vi "observacao_queued.vi"() -> ()   [LabVIEW 2012, in "Shared_160.lvlib"] (continued)
                    n1067 = call "Trata PDA.vi"() -> ()  [unwired: 2 in]
                  }
                  frame True {
                    n1068 = call "Find ppctxt.vi"() -> ("Existe ppc.txt?"=w1386:bool, "ppc.txt Path"=w1385:path)  [unwired: 1 in]
                    n1069 = case shown="True" w1386 {
                      tunnel: w1385 -> [_ w1387]
                      frame False {
                      }
                      frame True {
                        # "limpa o arquivo ppc.txt"
                        n1070 = call "Wipe file.vi"("ppc path"=w1387) -> ()  [unwired: 2 out]
                      }
                    }
                  }
                }
              }
              frame #1 {
                n1071 = case shown="False" "Case Constant\n(See Context Help) 3" {
                  frame False {
                  }
                  frame True {
                    # "MUDANÇA:\nÉ necesário \nsubstituir as variáveis simuladas pelas do Sistema"
                    # "Simula os dados sendo alterados pela\nmovimentação do sistema"
                    n1072 = call "Data Table.vi"() -> ()  [unwired: 1 in]
                  }
                }
              }
              frame #2 {
                n1073 = case shown="True" "Case Constant\n(See Context Help) 4" {
                  frame False {
                  }
                  frame True {
                    # "Lê o arquivo padrão para o equip/o\nselecionado pelo PDA e grava o\narquivo ppcDisplay.htm adequado"
                    n1074 = call "Update Frame.vi"() -> ("Timeout"=w1390:u32)  [unwired: 2 in, 3 out]
                    n1075 = Wait Until Next ms Multiple(millisecond multiple=w1390) -> ()  [unwired: 1 out]
                  }
                }
              }
            }
          }
        }
        n1076 = global read "Global_Telescopio.vi" "Flag-Rotator"() -> (w83:bool)
        n1077 = case shown="True" w83 {
          frame False {
          }
          frame True {
            n1078 = local write "Setup, Pointing & Guiding"(T2."ROTATOR" ("Setup, Pointing & Guiding")) -> ()
          }
        }
      }
      frame #2 {
        n1079 = case shown="\"FOCUS\"" "Setup, Pointing & Guiding" {
          frame "POINTING", Default {
            n1080 = stacked-sequence {
              frame #0 {
                # "Clear Dados"
                n1081 = case shown="True" "BtPointObjClear" {
                  frame False {
                  }
                  frame True {
                    w1395 = ""
                    n1082 = local write "StrPointObjName"(w1395) -> ()
                    n1083 = local write "StrPointObjPMRA"(w1395) -> ()
                    n1084 = local write "StrPointObjPMDEC"(w1395) -> ()
                    n1085 = local write "StrPointObjRA"(w1395) -> ()
                    n1086 = local write "StrPointObjDEC"(w1395) -> ()
                    n1087 = local write "StrPointObjEpoch"(w1395) -> ()
                    n1088 = local write "StrPointTargetRA"(w1395) -> ()
                    n1089 = local write "StrPointTargetDEC"(w1395) -> ()
                  }
                }
                n1090 = local read "ChkCalLocal"() -> (w1392:bool)
                n1091 = case shown="False" w1392 {
                  selector: w1392 -> [w1394 _]
                  frame False {
                    # "Para de Piscar/Blink\no botão"
                    n1092 = property on="ChkCalLocal" class="Bool (strict)"("Blinking"=w1394) -> ()  [unwired: 2 in, 2 out]
                  }
                  frame True {
                  }
                }
              }
              frame #1 {
                w1402 = ""
                # "A forma como os mostradores da janela TARGET são carregados está indefinida.\nVamos colocar um botão SET ao lado do botão CLEAR na janela OBJECT.\nQuando o botão SET for pressionado, os mostradores da janela TARGET\nseriam calculados a partir dos valores da janela OBJECT."
                n1093 = local read "StrPointObjDEC"() -> (w1403:string)
                n1094 = local read "StrPointObjRA"() -> (w1404:string)
                n1095 = local read "StrPointObjPMDEC"() -> (w1396:string)
                n1096 = local read "StrPointObjPMRA"() -> (w1397:string)
                n1097 = Not Equal?(x=w1404, y=w1402) -> (x != y?=w1401:bool)
                n1098 = Not Equal?(x=w1403, y=w1402) -> (x != y?=w1400:bool)
                n1099 = local read "pressão atm"() -> (w1406:string)
                n1100 = local read "Temp amb"() -> (w1407:string)
                n1101 = local read "hum local"() -> (w1405:string)
                n1102 = And(x=w1401, y=w1400) -> (x .and. y?=w1398:bool)
                n1103 = And(x="BtPointPrecess", y=w1398) -> (x .and. y?=w1399:bool)
                n1104 = case shown="True" w1399 {
                  tunnel: w1404 -> [_ w1415]
                  tunnel: w1403 -> [_ w1414]
                  tunnel: w1407 -> [_ w1413]
                  tunnel: w1406 -> [_ w1412]
                  tunnel: w1405 -> [_ w1411]
                  tunnel: w1397 -> [_ w1410]
                  tunnel: w1396 -> [_ w1409]
                  frame False {
                  }
                  frame True {
                    n1105 = stacked-sequence {
                      tunnel: w1415 -> [w1449 _ _]
                      tunnel: w1414 -> [w1447 _ _]
                      tunnel: w1413 -> [w1457 _ _]
                      tunnel: w1412 -> [w1456 _ _]
                      tunnel: w1411 -> [w1455 _ _]
                      tunnel: w1410 -> [w1423 _ _]
                      tunnel: w1409 -> [w1422 _ _]
                      frame #0 {
                        # "PROCESSO PRECESSÃO"
                        # "MUDANÇA:\nVI Botao SET trocada por Botao Precess, eliminando entrada do Frame de coord. (Mean, Topo, Geo)"
                        n1106 = local read "ChkPointPrecessed"() -> (w1427:bool)
                        n1107 = call "Comma_to_Point.vi"("Lat_A"=w1455) -> ("Saída"=w1424:string)
                        n1108 = call "Comma_to_Point.vi"("Lat_A"=w1457) -> ("Saída"=w1426:string)
                        n1109 = call "Comma_to_Point.vi"("Lat_A"=w1456) -> ("Saída"=w1425:string)
                        n1110 = call "Comma_to_Point.vi"("Lat_A"=w1447) -> ("Saída"=w1442:string)
                        n1111 = call "Comma_to_Point.vi"("Lat_A"=w1449) -> ("Saída"=w1445:string)
                        n1112 = call "hms_rad.vi"("True = hora"=FALSE, "Texto Graus"=w1442) -> ("radianos"=w1441:dbl)  [unwired: 3 in]
                        n1113 = call "hms_rad.vi"("True = hora"=TRUE, "Texto Graus"=w1445) -> ("radianos"=w1444:dbl)  [unwired: 3 in]
                        n1114 = call "Arcsec to Rad_ String.vi"("VAR ARCSEC"=w1423) -> ("VAR RAD"=w1421:string)
                        n1115 = Number To Fractional String(use system decimal point (T)=FALSE, number=w1441, precision (6)=i16 9) -> (F-format string=w1430:string)  [unwired: 1 in]
                        n1116 = Number To Fractional String(use system decimal point (T)=FALSE, number=w1444, precision (6)=i16 9) -> (F-format string=w1431:string)  [unwired: 1 in]
                        n1117 = call "Arcsec to Rad_ String.vi"("VAR ARCSEC"=w1422) -> ("VAR RAD"=w1420:string)
                        n1118 = call "Botão Precess.vi"("AR"=w1431, "Precessed Coord."=w1427, "Dec"=w1430, "Temp local amb(K)"=w1426, "Pressao atm local (mB)"=w1425, "Hum rel local"=w1424, "Var RA"=w1421, "Var DEC"=w1420) -> ("RA"=w1459:dbl, "DEC"=w1416:dbl, "Hora Sideral (rad)"=w1458:dbl, "Dist. Zenital (rad)"=w1429:dbl, "Observed HA (radians)"=→"HA obs":dbl, "Massa de Ar"=w1428:dbl)  [unwired: 2 in]
                        "RA obs" <- w1459
                        "DEC obs" <- w1416
                        n1119 = local write "Zenital angle"(w1429) -> ()
                        n1120 = call "rad_hms.vi"("TRUE=HORA\nFALSE=GRAU"=FALSE ("TRUE=HORA\nFALSE=GRAU"), "Radiano"=w1416) -> ("Hora/Graus Texto Decimal"=w1437:string)  [unwired: 3 in]
                        n1121 = call "rad-graus.vi"("Radiano"=w1429) -> ("Graus"=w1454:dbl)
                        n1122 = Number To Fractional String(number=w1428, precision (6)=i16 3) -> (F-format string=→"Air Mass":string)  [unwired: 2 in]
                        n1123 = Number To Fractional String(number=w1454, precision (6)=i16 1) -> (F-format string=→"Zenital Angle":string)  [unwired: 2 in]
                        n1124 = call "rad_hms.vi"("TRUE=HORA\nFALSE=GRAU"=TRUE ("TRUE=HORA"), "Radiano"=w1459) -> ("Hora/Graus Texto Decimal"=w1439:string)  [unwired: 3 in]
                        n1125 = local write "StrPointTargetDEC"(w1437) -> ()
                        n1126 = local write "StrPointTargetRA"(w1439) -> ()
                        n1127 = disable-structure shown="Disabled" {
                          disable-tunnel: [w1463 _] -> _
                          disable-tunnel: w1459 -> [w1462 _]
                          disable-tunnel: w1458 -> [w1461 _]
                          disable-tunnel: w1416 -> [w1460 _]
                          frame Disabled {
                            n1128 = call "Hora_Limite.vi"("Asc Reta RA rad"=w1462, "Sideral Time rad"=w1461, "Declinação rad"=w1460) -> ("TO Tempo de Observação Horas"=w1463:dbl)  [unwired: 2 in]
                          }
                          frame Enabled {
                          }
                        }
                        n1129 = call "Novo_tempo_obs_inicial.vi"("TS"=w1458, "RA"=w1459, "DEC"=w1416) -> ("TO rad"=w1417:dbl)  [unwired: 7 in, 1 out]
                        n1130 = case shown="True" "TRUE=HORA\nFALSE=GRAU" {
                          frame False {
                          }
                          frame True {
                            # "Sincroniza hora do\nPC com GPS"
                            n1131 = call "About_Time.vi"() -> ()  [unwired: 1 in]
                          }
                        }
                        n1132 = call "rad_hms.vi"("TRUE=HORA\nFALSE=GRAU"=TRUE ("TRUE=HORA\nFALSE=GRAU"), "Radiano"=w1417) -> ("Hora/Graus Texto Decimal"=→"Tempo Obs":string)  [unwired: 3 in]
                      }
                      frame #1 {
                        # "Testa o ângulo zenital menor que 70º o led \"Working Area\" \naceso na cor verde se o ângulozenital menor que 70º e \nvermelho em caso cont rário."
                        n1133 = global read "Global_Telescopio.vi" "Piscar working area"() -> (w1470:bool)
                        n1134 = global read "Global_Telescopio.vi" "working area = VERDE"() -> (w1469:bool)
                        n1135 = global read "Global_Telescopio.vi" "ativar botão GO"() -> (w1467:bool)
                        n1136 = case shown="True" w1469 {
                          frame False {
                            # "False=Vermelho"
                            n1137 = local write "LedPointWorkArea"(FALSE ("LedPointWorkArea")) -> ()
                          }
                          frame True {
                            # "True=Verde"
                            "LedPointWorkArea" <- TRUE ("LedPointWorkArea")
                          }
                        }
                        n1138 = global write "Global_Telescopio.vi" "Botão GO = STOP"(FALSE ("Botão GO = STOP")) -> ()
                        n1139 = case shown="True" w1467 {
                          selector: w1467 -> [_ w1471]
                          frame False {
                          }
                          frame True {
                            n1140 = property on="BtTargetPoint" class="Bool"("Visible"=w1471) -> ()  [unwired: 2 in, 2 out]
                          }
                        }
                        n1141 = global write "Global_Telescopio.vi" "Piscar working area"(w1470) -> ()
                        n1142 = global read "Global_Telescopio.vi" "desativar botão GO"() -> (w1468:bool)
                        n1143 = case shown="True" w1468 {
                          selector: w1468 -> [_ w1473]
                          frame False {
                          }
                          frame True {
                            n1144 = Not(x=w1473) -> (.not. x?=w1472:bool)
                            n1145 = property on="BtTargetPoint" class="Bool"("Visible"=w1472) -> ()  [unwired: 2 in, 2 out]
                          }
                        }
                        n1146 = property on="LedPointWorkArea" class="Bool (strict)"("Visible"=TRUE ("Botão GO = STOP")) -> ()  [unwired: 2 in, 2 out]
                        n1147 = property on="LedPointing" class="Bool (strict)"("Visible"=FALSE) -> ()  [unwired: 2 in, 2 out]
                      }
                      frame #2 {
                        n1148 = global read "Global_Telescopio.vi" "CalDEC Local"() -> (w1481:dbl)
                        n1149 = global read "Global_Telescopio.vi" "CalAH Local"() -> (w1482:dbl)
                        n1150 = local read "ChkCalLocal"() -> (w1476:bool)
                        n1151 = Not Equal To 0?(x=w1482) -> (x != 0?=w1479:bool)
                        n1152 = Not Equal To 0?(x=w1481) -> (x != 0?=w1480:bool)
                        n1153 = Or(x=w1479, y=w1480) -> (x .or. y?=w1477:bool)
                        n1154 = And(x=w1476, y=w1477) -> (x .and. y?=w1478:bool)
                        n1155 = case shown="True" w1478 {
                          frame False {
                          }
                          frame True {
                            n1156 = local read "HA obs"() -> (w1502:dbl)
                            n1157 = local read "DEC obs"() -> (w1496:dbl)
                            n1158 = global read "Global_Telescopio.vi" "AH Zero Local"() -> (w1500:dbl)
                            n1159 = global read "Global_Telescopio.vi" "DEC Zero Local"() -> (w1495:dbl)
                            n1160 = global read "Global_Telescopio.vi" "Raio Máximo"() -> (w1484:dbl)
                            n1161 = Cosine(x=w1496) -> (cos(x)=w1501:dbl)
                            n1162 = Cosine(x=w1495) -> (cos(x)=w1499:dbl)
                            n1163 = Multiply(x=w1502, y=w1501) -> (x*y=w1498:dbl)
                            n1164 = Multiply(x=w1500, y=w1499) -> (x*y=w1497:dbl)
                            n1165 = Subtract(x=w1496, y=w1495) -> (x-y=w1491:dbl)
                            n1166 = Multiply(x=w1491, y=w1491) -> (x*y=w1494:dbl)
                            n1167 = Subtract(x=w1498, y=w1497) -> (x-y=w1490:dbl)
                            n1168 = Multiply(x=w1490, y=w1490) -> (x*y=w1492:dbl)
                            n1169 = Add(x=w1492, y=w1494) -> (x+y=w1493:dbl)
                            n1170 = Square Root(x=w1493) -> (sqrt(x)=w1489:dbl)
                            n1171 = Multiply(x=w1489, y=180.0) -> (x*y=w1487:dbl)
                            n1172 = Divide(x=w1487, y=3.141592653589793) -> (x/y=w1485:dbl)
                            n1173 = Greater?(x=w1485, y=w1484) -> (0:w1483:bool)
                            n1174 = property on="ChkCalLocal" class="Bool (strict)"("Blinking"=w1483) -> ()  [unwired: 2 in, 2 out]
                          }
                        }
                      }
                    }
                  }
                }
              }
              frame #2 {
                # "Clicando-se essa Tecla\nInicia-se o Apontamento"
                n1175 = local read "StrPointObjRA"() -> (w1513:string)
                n1176 = local read "StrPointObjDEC"() -> (w1512:string)
                n1177 = local read "StrPointObjPMDEC"() -> (w1504:string)
                n1178 = local read "pressão atm"() -> (w1505:string)
                n1179 = local read "hum local"() -> (w1511:string)
                n1180 = local read "StrPointObjPMRA"() -> (w1503:string)
                n1181 = local read "Temp amb"() -> (w1506:string)
                n1182 = control-ref of="BtTargetPoint"() -> (w1508:refnum<vi>)
                n1183 = property class="Bool"(reference=w1508) -> ("Boolean Text.Text"=w1509:string)  [unwired: 1 in, 2 out]
                n1184 = Equal?(x=w1509, y="POINT") -> (x = y?=w1507:bool)
                n1185 = case shown="True" "BtTargetPoint" {
                  tunnel: w1513 -> [_ w1519]
                  tunnel: w1512 -> [_ w1523]
                  tunnel: w1506 -> [_ w1520]
                  tunnel: w1505 -> [_ w1521]
                  tunnel: w1511 -> [_ w1522]
                  tunnel: w1507 -> [_ w1517]
                  tunnel: w1504 -> [_ w1516]
                  tunnel: w1503 -> [_ w1515]
                  frame False {
                  }
                  frame True {
                    n1186 = case shown="True" w1517 {
                      selector: w1517 -> [w1525 _]
                      tunnel: w1523 -> [_ w1555]
                      tunnel: w1522 -> [_ w1535]
                      tunnel: w1521 -> [_ w1534]
                      tunnel: w1520 -> [_ w1533]
                      tunnel: w1519 -> [_ w1554]
                      tunnel: w1516 -> [_ w1549]
                      tunnel: w1515 -> [_ w1550]
                      frame False {
                        w1526 = 0 ("estado")
                        # "Zera Máquina de Estado\nPelo Botão STOP"
                        n1187 = Not(x=w1525) -> (.not. x?=w1527:bool)
                        n1188 = local write "LedPointing"(w1525) -> ()
                        n1189 = global write "Global_Telescopio.vi" "Botão GO = STOP"(w1527) -> ()
                        n1190 = call "Stop.vi"() -> ()  [unwired: 1 in, 1 out]
                        n1191 = local write "statDEC"(w1526) -> ()
                        n1192 = local write "statAH"(w1526) -> ()
                        n1193 = local write "statCUP"(w1526) -> ()
                        "Flag Stop" <- TRUE ("Flag Stop")
                      }
                      frame True {
                        w1528 = ""
                        w1553 = FALSE ("use system decimal point (T)")
                        n1194 = call "Comma_to_Point.vi"("Lat_A"=w1554) -> ("Saída"=w1543:string)
                        n1195 = call "Comma_to_Point.vi"("Lat_A"=w1555) -> ("Saída"=w1544:string)
                        n1196 = call "Arcsec to Rad_ String.vi"("VAR ARCSEC"=w1550) -> ("VAR RAD"=w1531:string)
                        n1197 = call "hms_rad.vi"("True = hora"=TRUE, "Texto Graus"=w1543) -> ("radianos"=w1558:dbl)  [unwired: 3 in]
                        n1198 = call "hms_rad.vi"("True = hora"=FALSE, "Texto Graus"=w1544) -> ("radianos"=w1556:dbl)  [unwired: 3 in]
                        n1199 = call "Arcsec to Rad_ String.vi"("VAR ARCSEC"=w1549) -> ("VAR RAD"=w1532:string)
                        n1200 = local write "NAME"(w1528) -> ()
                        n1201 = local write "RA"(w1528) -> ()
                        n1202 = local write "DEC"(w1528) -> ()
                        n1203 = Number To Fractional String(use system decimal point (T)=w1553, number=w1558, precision (6)=i16 9) -> (F-format string=w1530:string)  [unwired: 1 in]
                        n1204 = Number To Fractional String(use system decimal point (T)=w1553, number=w1556, precision (6)=i16 9) -> (F-format string=w1529:string)  [unwired: 1 in]
                        n1205 = Concatenate Strings("Apontamento:" ("string"), "RA= " ("string"), w1543, " " ("string"), "DEC= " ("string"), w1544) -> ()  [unwired: 1 out]
                        n1206 = call "PrecessaoCorrigida.vi"("Coordenada do dia"="ChkPointPrecessed", "HabCorrModelo"="ChkModel", "UseLocalZero"="ChkCalLocal", "UseGlobalZero"="ChkCalGlobal", "RA"=w1530, "DEC"=w1529, "MovProprioRA"=w1531, "MovProprioDEC"=w1532, "Temp amb (K)"=w1533, "Press atm (mB)"=w1534, "Humid relat"=w1535) -> ("Estado"=w1538:i32, "RA"=w1537:dbl, "DEC"=w1536:dbl)  [unwired: 2 out]
                        n1207 = Equal To 0?(x=w1538) -> (x = 0?=w1551:bool)
                        n1208 = case shown="False" w1551 {
                          selector: w1551 -> [w1574 _]
                          tunnel: "ChkCalLocal" -> [w1586 _]
                          tunnel: "ChkCalGlobal" -> [w1585 _]
                          tunnel: w1529 -> [w1584 _]
                          tunnel: w1530 -> [w1583 _]
                          tunnel: w1532 -> [w1580 _]
                          tunnel: w1531 -> [w1579 _]
                          tunnel: w1538 -> [w1561 _]
                          tunnel: w1537 -> [w1582 _]
                          tunnel: w1536 -> [w1581 _]
                          tunnel: "ChkPointPrecessed" -> [w1577 _]
                          frame False {
                            w1564 = FALSE ("Coude")
                            w1565 = FALSE ("WeakSel")
                            w1566 = T5."Enabled" ("Disabled")
                            w1567 = TRUE ("MOUNT")
                            w1578 = 0 ("M_AH")
                            w1575 = TRUE
                            # "ABAS DE CONTROLE"
                            # "MUDANÇA:\nIncluído CASE"
                            # "Seta máquinas de\nestado aba ÚTILS"
                            n1209 = global write "Global_Telescopio.vi" "CoordDia"(w1577) -> ()
                            n1210 = global write "Global_Telescopio.vi" "CalGlobal"(w1585) -> ()
                            n1211 = global write "Global_Telescopio.vi" "CalLocal"(w1586) -> ()
                            n1212 = call "Envia LOG.vi"() -> ()  [unwired: 8 in, 2 out]
                            n1213 = global write "Global_Telescopio.vi" "TargetRA"(w1582) -> ()
                            n1214 = global write "Global_Telescopio.vi" "TargetDEC"(w1581) -> ()
                            n1215 = local write "statAH"(w1561) -> ()
                            n1216 = property on="LedPointWorkArea" class="Bool (strict)"("Visible"=FALSE ("Botão GO = STOP")) -> ()  [unwired: 2 in, 2 out]
                            n1217 = local write "statDEC"(w1561) -> ()
                            n1218 = global write "Global_Telescopio.vi" "ObjCentrado"(w1574) -> ()
                            n1219 = local write "RA on Target"(w1574) -> ()
                            n1220 = local write "DEC on Target"(w1574) -> ()
                            n1221 = local write "Dome on Target"(w1574) -> ()
                            n1222 = local read "ChkDomeEnable"() -> (w1573:bool)
                            n1223 = local write "M_AH"(w1578) -> ()
                            n1224 = local write "M_DEC"(w1578) -> ()
                            n1225 = local write "M_CUP"(w1578) -> ()
                            n1226 = case shown="False" w1573 {
                              selector: w1573 -> [w1607 _]
                              tunnel: w1561 -> [_ w1609]
                              tunnel: [0 ("Estado") w1609] -> w1572
                              tunnel: [u8 2 ("Disabled") u8 0 ("Disabled")] -> w1571
                              frame False {
                                n1227 = local write "DOME"(w1607) -> ()
                              }
                              frame True {
                              }
                            }
                            n1228 = Tick Count (ms)() -> (millisecond timer value=w1569:u32)
                            n1229 = Add(x=w1569, y=u32 120000) -> (x+y=w1570:u32)
                            n1230 = local write "Tick Cupula"(w1570) -> ()
                            n1231 = local write "GUIDER"(w1567) -> ()
                            n1232 = local write "MOUNT"(w1567) -> ()
                            n1233 = property on="LedPointing" class="Bool (strict)"("Visible"=w1575) -> ()  [unwired: 2 in, 2 out]
                            n1234 = local write "statCUP"(w1572) -> ()
                            n1235 = property on="DOME" class="Bool (strict)"("Disabled"=w1571) -> ()  [unwired: 2 in, 2 out]
                            n1236 = stacked-sequence {
                              frame #0 {
                                n1237 = local read "StrPointObjName"() -> (w1587:string)
                                n1238 = local read "StrPointObjRA"() -> (w1588:string)
                                n1239 = local read "StrPointObjDEC"() -> (w1589:string)
                                n1240 = global write "Global_Telescopio.vi" "RA AUX"(w1588) -> ()
                                n1241 = global write "Global_Telescopio.vi" "DEC AUX"(w1589) -> ()
                                n1242 = global write "Global_Telescopio.vi" "NAME OBJETO AUX"(w1587) -> ()
                              }
                              frame #1 {
                                w1591 = u16 4 items=["ZERO", "AH", "DEC", "TUBO", "CUP"] ("Controlador")
                                n1243 = call "Monta Comando.vi"("Comando"="DESLIGAR", "Dispositivo"="FLAT_WEAK", "Controlador"=w1591) -> ()  [unwired: 4 in, 3 out]
                              }
                              frame #2 {
                                w1594 = u16 4 items=["ZERO", "AH", "DEC", "TUBO", "CUP"] ("Controlador")
                                n1244 = call "Monta Comando.vi"("Comando"="DESLIGAR", "Dispositivo"="FLAT_LO", "Controlador"=w1594) -> ()  [unwired: 4 in, 3 out]
                              }
                              frame #3 {
                                w1597 = u16 4 items=["ZERO", "AH", "DEC", "TUBO", "CUP"] ("Controlador")
                                n1245 = call "Monta Comando.vi"("Comando"="DESLIGAR", "Dispositivo"="FLAT_HI", "Controlador"=w1597) -> ()  [unwired: 4 in, 3 out]
                              }
                              frame #4 {
                                w1599 = u16 4 items=["ZERO", "AH", "DEC", "TUBO", "CUP"] ("Controlador")
                                n1246 = call "Monta Comando.vi"("Comando"="DESLIGAR", "Dispositivo"="FLAT_COUDE", "Controlador"=w1599) -> ()  [unwired: 4 in, 3 out]
                              }
                              frame #5 {
                                w1602 = u16 4 items=["ZERO", "AH", "DEC", "TUBO", "CUP"] ("Controlador")
                                n1247 = call "Monta Comando.vi"("Comando"="LIGAR", "Dispositivo"="LAMP_CAM", "Controlador"=w1602) -> ()  [unwired: 4 in, 3 out]
                              }
                              frame #6 {
                                n1248 = call "Log_Apontamento.vi"() -> ()  [unwired: 12 in]
                              }
                            }
                            n1249 = local write "WeakSel"(w1565) -> ()
                            n1250 = local write "MediumSel"(w1565) -> ()
                            n1251 = local write "StrongSel"(w1565) -> ()
                            n1252 = local write "CoudeSel"(w1565) -> ()
                            n1253 = local write "Coude"(w1564) -> ()
                            n1254 = local write "Weak"(w1564) -> ()
                            n1255 = local write "Medium"(w1564) -> ()
                            n1256 = local write "Strong"(w1564) -> ()
                            n1257 = local write "DOME"(FALSE ("WeakSel")) -> ()
                            n1258 = property on="Medium" class="Bool (strict)"("Disabled"=w1566) -> ()  [unwired: 2 in, 2 out]
                            n1259 = property on="Strong" class="Bool (strict)"("Disabled"=w1566) -> ()  [unwired: 2 in, 2 out]
                            n1260 = property on="Coude" class="Bool (strict)"("DisabledEnum"=w1566) -> ()  [unwired: 2 in, 2 out]
                            n1261 = property on="Weak" class="Bool (strict)"("Disabled"=w1566) -> ()  [unwired: 2 in, 2 out]
                            "MeanDEC" <- w1584
                            "MeanRA" <- w1583
                            "LedPointing" <- w1575
                            "PM_DEC" <- w1580
                            "PM_RA" <- w1579
                            "Apontou" <- TRUE ("WeakSel")
                          }
                          frame True {
                          }
                        }
                      }
                    }
                    n1262 = property on="Delete Calagem" class="Bool"("Disabled"=u8 0) -> ()  [unwired: 2 in, 2 out]
                  }
                }
              }
              frame #3 {
                # "e o led \"Working Area\" aceso na cor verde se o ângulo\nzenital menor que 70º e vermelho em caso cont rário.\nO botão GO ao ser clicado dispara o apontamento virtual do telescópio. Caso esse\nbotão seja pressionado enquanto o led \"Working Area\" est iver vermelho, este deve\npiscar 3 vezes e nada mais é executado. Caso cont rário, o nome do botão GO passa\npara CANCEL e o led \"Mount in Posit ion\" da janela STATUS INFORMATION deve ser\ndesligado, o que provocará a simulação do apontamento do telescópio (cf. item 4.3) .\nOs valores dos comandos \"Epoch\" , \"RA Proper Mot ion\" e \"DEC Proper Mot ion\" desse\nquadro devem ser ignorados na simulação."
                # "Habilita Cancela"
                # "Habilita Apontamento"
                n1263 = case shown="True" "Case Constant\n(See Context Help) 5" {
                  frame False {
                  }
                  frame True {
                    w1615 = TRUE ("Go aux")
                    w1616 = ""
                    n1264 = local write "LED MOUNT"(w1615) -> ()
                    n1265 = local write "MOUNT"(w1615) -> ()
                    n1266 = control-ref of="BtTargetPoint"() -> (w1617:refnum<vi>)
                    n1267 = local write "DEC"(w1616) -> ()
                    n1268 = local write "RA"(w1616) -> ()
                    n1269 = local write "NAME"(w1616) -> ()
                    n1270 = property class="Bool"(reference=w1617, "Boolean Text.Text"="STOP") -> ()  [unwired: 1 in, 2 out]
                  }
                }
                n1271 = case shown="True" "Case Constant\n(See Context Help) 6" {
                  frame False {
                  }
                  frame True {
                    w1612 = FALSE ("Go aux")
                    # "Seta nome para GO"
                    n1272 = local write "LED MOUNT"(w1612) -> ()
                    n1273 = local write "MOUNT"(w1612) -> ()
                    n1274 = control-ref of="BtTargetPoint"() -> (w1613:refnum<vi>)
                    n1275 = property class="Bool"(reference=w1613, "Boolean Text.Text"="POINT") -> ()  [unwired: 1 in, 2 out]
                  }
                }
              }
              frame #4 {
                # "Detecta Edição"
                # "os valores de RA e DEC devem assumir os valores da janela OBJECT da aba POINTING ao TÉRMINO do apontamento. Durante o apontamento devem ficar apagados. Como o campo MAG daquela janela não tem um valor correspondente na janela OBJECT, o campo MAG deve ficar em branco. Apenas quando as coordenadas da janela OBJECT da aba POINTING forem preenchidos a partir do botão SET COORD da aba LIST é que o campo MAG da janela TARGET assume o valor da coluna MAG da aba LIST. Colocar um flag interno (invisível para o usuário) para definir se o campo MAG deve ou não ser preenchido com o valor da aba LIST. Quando o botão SET COORD. fosse pressionado esse flag assumiria o valor verdadeiro e caso ocorresse edição dos valores da janela \nOBJECT da aba POINTING, esse flag assumiria o valor falso e o campo MAG da janela TARGET (entre os controles das abas e as imagens) ficaria vazio durante e após o apontamento"
                n1276 = local read "StrPointObjPMRA"() -> (w1632:string)
                n1277 = local read "StrPointObjPMDEC"() -> (w1631:string)
                n1278 = local read "StrPointObjName"() -> (w1639:string)
                n1279 = local read "AUX EDITA Name"() -> (w1638:string)
                n1280 = local read "StrPointObjEpoch"() -> (w1633:string)
                n1281 = local read "AUX EDITA PMDEC"() -> (w1630:string)
                n1282 = local read "StrPointObjRA"() -> (w1637:string)
                n1283 = local read "StrPointObjDEC"() -> (w1635:string)
                n1284 = local read "AUX EDITA EPOCH"() -> (w1628:string)
                n1285 = local read "AUX EDITA PMRA"() -> (w1629:string)
                n1286 = local read "AUX EDITA DEC"() -> (w1634:string)
                n1287 = local read "AUX EDITA RA"() -> (w1636:string)
                n1288 = Not Equal?(x=w1632, y=w1629) -> (x != y?=w1623:bool)
                n1289 = Not Equal?(x=w1639, y=w1638) -> (x != y?=w1627:bool)
                n1290 = Not Equal?(x=w1633, y=w1628) -> (x != y?=w1624:bool)
                n1291 = Not Equal?(x=w1631, y=w1630) -> (x != y?=w1622:bool)
                n1292 = Not Equal?(x=w1637, y=w1636) -> (x != y?=w1626:bool)
                n1293 = Not Equal?(x=w1635, y=w1634) -> (x != y?=w1625:bool)
                n1294 = Compound Arithmetic op=OR(w1627, w1626, w1625, w1624, w1623, w1622) -> (w1619:bool)
                n1295 = local read "FLAG SET COORD"() -> (w1620:bool)
                n1296 = And(x=w1619, y=w1620) -> (x .and. y?=w1621:bool)
                n1297 = case shown="True" w1621 {
                  frame False {
                  }
                  frame True {
                    # "Se houver edição o flag é resetado"
                    n1298 = local write "MAG"("") -> ()
                    "FLAG SET COORD" <- FALSE ("FLAG SET ACOORD")
                  }
                }
              }
            }
          }
          frame "HANDSET" {
            # "PROCESSO DISPLAY DESLOCAMENTO"
            n1299 = local read "AtualDEC"() -> (w1655:dbl)
            n1300 = global read "Global_Telescopio.vi" "Sideral Time"() -> (w1648:dbl)
            n1301 = global read "Global_Telescopio.vi" "PosAH"() -> (w1646:dbl)
            n1302 = Multiply(x="Velocity (arcsec/sec)", y=100.0) -> (x*y=w1663:dbl)
            n1303 = Cosine(x=w1655) -> (cos(x)=w1654:dbl)
            n1304 = Subtract(x=w1648, y=w1646) -> (x-y=w1647:dbl)
            n1305 = Absolute Value(x=w1654) -> (abs(x)=w1651:dbl)
            n1306 = Add(x=1e-10, y=w1651) -> (x+y=w1653:dbl)
            n1307 = local read "LatchDeslocRA"() -> (w1659:dbl)
            n1308 = local read "LatchDeslocDEC"() -> (w1658:dbl)
            n1309 = global read "Global_Telescopio.vi" "PosDEC"() -> (w1649:dbl)
            n1310 = event shown="[9] \"Calagem\": Value Change" {
              selector: _ -> [_ _ _ _ _ _ _ _ _ _ _]
              dyn-events: _ -> [_ _ _ _ _ _ _ _ _ _ _]
              timeout: 10 -> [_ _ _ _ _ _ _ _ _ _ _]
              tunnel: w1663 -> [_ w1676 w1684 w1692 _ _ _ _ _ _ w1795]
              tunnel: "Global" -> [_ _ _ _ _ _ _ _ w1737 w1757 _]
              tunnel: w1647 -> [_ _ _ _ w1695 _ _ _ _ w1755 _]
              tunnel: w1649 -> [_ _ _ _ _ w1696 _ _ _ w1756 _]
              tunnel: w1653 -> [_ _ _ _ _ _ w1697 w1715 _ _ _]
              event Timeout {
                n1311 = event-data() -> ()  [unwired: 1 in, 2 out]
              }
              event "Left HS": Value Change {
                w1673 = u8 0 ("Disabled")
                n1312 = event-data() -> ("NewVal"=w1672:bool)  [unwired: 1 in, 5 out]
                "MOV_IDX_AH" <- w1672
                n1313 = Select(t=u8 2 ("Disabled"), s=FALSE, f=w1673) -> (s? t:f=w1674:u8)
                n1314 = call "Tx handeset.vi"("CMD On"="left" ("Comando"), "CMD Off"="stoph" ("Comando"), "Estado do Botão"=w1672, "Velocity (arcsec/sec)"=w1676) -> ()  [unwired: 12 in]
                n1315 = property on="Delete Calagem" class="Bool"("Disabled"=w1673) -> ()  [unwired: 2 in, 2 out]
                n1316 = property on="Right HS" class="Bool (strict)"("Disabled"=w1674) -> ()  [unwired: 2 in, 2 out]
              }
              event "Down HS": Value Change {
                w1680 = u8 0 ("Disabled")
                n1317 = event-data() -> ("NewVal"=w1683:bool)  [unwired: 1 in, 5 out]
                "MOV_IDX_DEC" <- w1683
                n1318 = call "Tx handeset.vi"("CMD On"="down" ("Comando"), "CMD Off"="stopv" ("Comando"), "Estado do Botão"=w1683, "Velocity (arcsec/sec)"=w1684) -> ()  [unwired: 12 in]
                n1319 = Select(t=u8 2 ("Disabled"), s=FALSE, f=w1680) -> (s? t:f=w1681:u8)
                n1320 = property on="Delete Calagem" class="Bool"("Disabled"=w1680) -> ()  [unwired: 2 in, 2 out]
                n1321 = property on="Up HS" class="Bool (strict)"("Disabled"=w1681) -> ()  [unwired: 2 in, 2 out]
              }
              event "Right HS": Value Change {
                w1689 = u8 0 ("Disabled")
                n1322 = event-data() -> ("NewVal"=w1688:bool)  [unwired: 1 in, 5 out]
                n1323 = call "Tx handeset.vi"("CMD On"="right" ("Comando"), "CMD Off"="stoph" ("Comando"), "Estado do Botão"=w1688, "Velocity (arcsec/sec)"=w1692) -> ()  [unwired: 12 in]
                n1324 = Select(t=u8 2 ("Disabled"), s=FALSE, f=w1689) -> (s? t:f=w1690:u8)
                n1325 = property on="Delete Calagem" class="Bool"("Disabled"=w1689) -> ()  [unwired: 2 in, 2 out]
                n1326 = local write "MOV_IDX_AH"(w1688) -> ()
                n1327 = property on="Left HS" class="Bool (strict)"("Disabled"=w1690) -> ()  [unwired: 2 in, 2 out]
              }
              event "ClearDeslocRA": Value Change {
                n1328 = event-data() -> ()  [unwired: 1 in, 6 out]
                "LatchDeslocRA" <- w1695
              }
              event "ClearDeslocDEC": Value Change {
                n1329 = event-data() -> ()  [unwired: 1 in, 6 out]
                "LatchDeslocDEC" <- w1696
              }
              event "BtPrecCentrar": Value Change {
                # "PROCESSO OFFSET"
                n1330 = event-data() -> ()  [unwired: 1 in, 6 out]
                n1331 = stacked-sequence {
                  tunnel: w1697 -> [_ w1706]
                  frame #0 {
                    n1332 = local read "Offset DEC"() -> (w1698:dbl)
                    n1333 = Negate(x=w1698) -> (-x=w1699:dbl)
                    n1334 = Equal To 0?(x=w1698) -> (x = 0?=w1700:bool)
                    n1335 = case shown="False" w1700 {
                      tunnel: w1699 -> [w1701 _]
                      frame False {
                        n1336 = call "Conversao Ms to Hora texto.vi"("TRUE=HORA\nFALSE=GRAU"=FALSE ("TRUE=HORA\nFALSE=GRAU"), "PrecDEC"=w1701) -> ("Hora/Graus Texto Decimal"=w1703:string)
                        n1337 = call "Tx handeset.vi"("CMD On"="goDEC", "Set Point"=w1703, "Estado do Botão"=TRUE ("TRUE=HORA\nFALSE=GRAU")) -> ()  [unwired: 13 in]
                      }
                      frame True {
                      }
                    }
                  }
                  frame #1 {
                    # "PROCESSO MOVE TELESCÓPIO"
                    n1338 = local read "Offset RA"() -> (w1707:dbl)
                    n1339 = Equal To 0?(x=w1707) -> (x = 0?=w1708:bool)
                    n1340 = case shown="False" w1708 {
                      tunnel: w1707 -> [w1710 _]
                      tunnel: w1706 -> [w1709 _]
                      frame False {
                        w1712 = TRUE ("TRUE=HORA\nFALSE=GRAU")
                        # "AH tem sentido\ncontrário de RA"
                        n1341 = Divide(x=w1710, y=w1709) -> (x/y=w1711:dbl)
                        n1342 = call "Conversao Ms to Hora texto.vi"("TRUE=HORA\nFALSE=GRAU"=w1712, "PrecDEC"=w1711) -> ("Hora/Graus Texto Decimal"=w1713:string)
                        n1343 = call "Tx handeset.vi"("CMD On"="goRA", "Set Point"=w1713, "Estado do Botão"=w1712) -> ()  [unwired: 13 in]
                      }
                      frame True {
                      }
                    }
                  }
                }
              }
              event "BtPrecGO": Value Change {
                # "PROCESSO OFFSET"
                n1344 = event-data() -> ("NewVal"=w1717:bool)  [unwired: 1 in, 5 out]
                n1345 = case shown="True" w1717 {
                  tunnel: w1715 -> [_ w1718]
                  frame False {
                  }
                  frame True {
                    # "PROCESSO MOVE TELESCÓPIO"
                    n1346 = stacked-sequence {
                      tunnel: w1718 -> [_ w1726]
                      frame #0 {
                        n1347 = Not Equal To 0?(x="PreciseOffsetDEC") -> (x != 0?=w1720:bool)
                        n1348 = case shown="True" w1720 {
                          tunnel: "PreciseOffsetDEC" -> [_ w1721]
                          frame False {
                          }
                          frame True {
                            n1349 = call "Conversao Ms to Hora texto.vi"("TRUE=HORA\nFALSE=GRAU"=FALSE ("TRUE=HORA\nFALSE=GRAU"), "PrecDEC"=w1721) -> ("Hora/Graus Texto Decimal"=w1723:string)
                            n1350 = call "Tx handeset.vi"("CMD On"="goDEC", "Set Point"=w1723, "Estado do Botão"=TRUE ("TRUE=HORA\nFALSE=GRAU")) -> ()  [unwired: 13 in]
                          }
                        }
                      }
                      frame #1 {
                        n1351 = Not Equal To 0?(x="PreciseOffsetRA") -> (x != 0?=w1729:bool)
                        n1352 = Negate(x="PreciseOffsetRA") -> (-x=w1728:dbl)
                        n1353 = case shown="True" w1729 {
                          tunnel: w1728 -> [_ w1731]
                          tunnel: w1726 -> [_ w1730]
                          frame False {
                          }
                          frame True {
                            n1354 = Divide(x=w1731, y=w1730) -> (x/y=w1732:dbl)
                            n1355 = call "Conversao Ms to Hora texto.vi"("TRUE=HORA\nFALSE=GRAU"=TRUE ("TRUE=HORA\nFALSE=GRAU"), "PrecDEC"=w1732) -> ("Hora/Graus Texto Decimal"=w1734:string)
                            n1356 = call "Tx handeset.vi"("CMD On"="goRA", "Set Point"=w1734, "Estado do Botão"=TRUE ("TRUE=HORA\nFALSE=GRAU")) -> ()  [unwired: 13 in]
                          }
                        }
                      }
                    }
                  }
                }
                n1357 = property on="Delete Calagem" class="Bool"("Disabled"=u8 2) -> ()  [unwired: 2 in, 2 out]
              }
              event "Delete Calagem": Value Change {
                n1358 = event-data() -> ()  [unwired: 1 in, 6 out]
                n1359 = case shown="True" w1737 {
                  tunnel: 0.0 ("Calagem DEC Rel") -> [w1739 w1740]
                  frame False {
                    # "Local"
                    n1360 = global write "Global_Telescopio.vi" "CalAH Local"(w1739) -> ()
                    n1361 = global write "Global_Telescopio.vi" "CalDEC Local"(w1739) -> ()
                  }
                  frame True {
                    # "Global"
                    n1362 = global write "Global_Telescopio.vi" "Calagem AH"(w1740) -> ()
                    n1363 = global write "Global_Telescopio.vi" "Calagem DEC"(w1740) -> ()
                  }
                }
              }
              event "Calagem": Value Change {
                # "PROCESSO CALAGEM"
                n1364 = event-data() -> ()  [unwired: 1 in, 6 out]
                n1365 = local read "ChkModel"() -> (w1746:bool)
                n1366 = local read "Temp amb"() -> (w1750:string)
                n1367 = local read "hum local"() -> (w1752:string)
                n1368 = local read "MeanDEC"() -> (w1743:string)
                n1369 = local read "MeanRA"() -> (w1747:string)
                n1370 = local read "PM_RA"() -> (w1748:string)
                n1371 = local read "PM_DEC"() -> (w1749:string)
                n1372 = local read "pressão atm"() -> (w1751:string)
                n1373 = global read "Global_Telescopio.vi" "CalGlobal"() -> (w1744:bool)
                n1374 = global read "Global_Telescopio.vi" "CalLocal"() -> (w1745:bool)
                n1375 = global read "Global_Telescopio.vi" "CoordDia"() -> (w1742:bool)
                n1376 = call "PrecessaoCorrigida.vi"("Coordenada do dia"=w1742, "HabCorrModelo"=w1746, "UseLocalZero"=w1745, "UseGlobalZero"=w1744, "RA"=w1747, "DEC"=w1743, "MovProprioRA"=w1748, "MovProprioDEC"=w1749, "Temp amb (K)"=w1750, "Press atm (mB)"=w1751, "Humid relat"=w1752) -> ("RA"=w1754:dbl, "DEC"=w1753:dbl, "AH"=w1741:dbl)  [unwired: 2 out]
                n1377 = case shown="True" w1757 {
                  tunnel: w1754 -> [w1767 w1770]
                  tunnel: w1753 -> [w1759 w1772]
                  tunnel: w1756 -> [w1766 w1773]
                  tunnel: w1755 -> [w1768 w1771]
                  tunnel: w1741 -> [w1758 _]
                  frame False {
                    # "Local"
                    n1378 = Subtract(x=w1768, y=w1767) -> (x-y=w1769:dbl)
                    n1379 = Subtract(x=w1766, y=w1759) -> (x-y=w1763:dbl)
                    n1380 = global read "Global_Telescopio.vi" "CalAH Local"() -> (w1762:dbl)
                    n1381 = global read "Global_Telescopio.vi" "CalDEC Local"() -> (w1764:dbl)
                    n1382 = global write "Global_Telescopio.vi" "AH Zero Local"(w1758) -> ()
                    n1383 = global write "Global_Telescopio.vi" "DEC Zero Local"(w1759) -> ()
                    n1384 = Negate(x=w1769) -> (-x=w1765:dbl)
                    n1385 = Add(x=w1765, y=w1762) -> (x+y=w1761:dbl)
                    n1386 = Add(x=w1763, y=w1764) -> (x+y=w1760:dbl)
                    n1387 = global write "Global_Telescopio.vi" "CalAH Local"(w1761) -> ()
                    n1388 = global write "Global_Telescopio.vi" "CalDEC Local"(w1760) -> ()
                  }
                  frame True {
                    # "Global"
                    n1389 = stacked-sequence {
                      tunnel: w1773 -> [w1783 _ _]
                      tunnel: w1772 -> [w1782 _ _]
                      tunnel: w1771 -> [w1778 _ _]
                      tunnel: w1770 -> [w1777 _ _]
                      frame #0 {
                        w1774 = 0.0 ("CalAH Local")
                        n1390 = Subtract(x=w1778, y=w1777) -> (x-y=w1776:dbl)
                        n1391 = Subtract(x=w1783, y=w1782) -> (x-y=w1784:dbl)
                        n1392 = global read "Global_Telescopio.vi" "Calagem AH"() -> (w1781:dbl)
                        n1393 = global read "Global_Telescopio.vi" "Calagem DEC"() -> (w1786:dbl)
                        n1394 = Negate(x=w1776) -> (-x=w1779:dbl)
                        n1395 = local write "Processa Centragem"(TRUE) -> ()
                        n1396 = Add(x=w1779, y=w1781) -> (x+y=w1780:dbl)
                        n1397 = Add(x=w1784, y=w1786) -> (x+y=w1785:dbl)
                        n1398 = global write "Global_Telescopio.vi" "Calagem AH"(w1780) -> ()
                        n1399 = global write "Global_Telescopio.vi" "CalAH Local"(w1774) -> ()
                        n1400 = global write "Global_Telescopio.vi" "CalDEC Local"(w1774) -> ()
                        n1401 = global write "Global_Telescopio.vi" "Calagem DEC"(w1785) -> ()
                      }
                      frame #1 {
                        # "25/10/2012 - Sempre que o usuario faz uma \ncalagem global, o valor da calagem e'  salva \nautomaticamente em GLOBAIS_CALAGEM.DAT"
                        n1402 = call "Salva_Calagem_Global.vi"() -> ()  [unwired: 1 in]
                      }
                      frame #2 {
                        # "Salva no Logo valor \ndo deslocamento da \ncalagem global"
                        n1403 = local read "DeslocDEC"() -> (w1787:dbl)
                        n1404 = local read "DeslocRA"() -> (w1788:dbl)
                        n1405 = call "Log_Calagem.vi"("Desloc DEC"=w1787, "Desloc RA"=w1788, "File Name"="LOG_COMANDOS.TXT") -> ()  [unwired: 3 in]
                      }
                    }
                  }
                }
              }
              event "Up HS": Value Change {
                w1792 = u8 0 ("Disabled")
                n1406 = event-data() -> ("NewVal"=w1791:bool)  [unwired: 1 in, 5 out]
                n1407 = call "Tx handeset.vi"("CMD On"="up" ("Comando"), "CMD Off"="stopv" ("Comando"), "Estado do Botão"=w1791, "Velocity (arcsec/sec)"=w1795) -> ()  [unwired: 12 in]
                n1408 = property on="Delete Calagem" class="Bool"("Disabled"=w1792) -> ()  [unwired: 2 in, 2 out]
                n1409 = Select(t=u8 2 ("Disabled"), s=FALSE, f=w1792) -> (s? t:f=w1793:u8)
                n1410 = local write "MOV_IDX_DEC"(w1791) -> ()
                n1411 = property on="Down HS" class="Bool (strict)"("Disabled"=w1793) -> ()  [unwired: 2 in, 2 out]
              }
            }
            n1412 = Subtract(x=w1647, y=w1659) -> (x-y=w1656:dbl)
            n1413 = Subtract(x=w1649, y=w1658) -> (x-y=w1660:dbl)
            n1414 = Multiply(x=w1656, y=w1653) -> (x*y=w1657:dbl)
            n1415 = global read "Global_Telescopio.vi" "ObjCentrado"() -> (w1650:bool)
            n1416 = call "Rad to Arcsec.vi"("Radiano"=w1657) -> ("Arcsec"=w1643:dbl)
            n1417 = call "Rad to Arcsec.vi"("Radiano"=w1660) -> ("Arcsec"=w1642:dbl)
            n1418 = case shown="False" w1650 {
              tunnel: [w1666 w1668] -> w1645
              tunnel: [w1666 w1669] -> w1644
              tunnel: w1643 -> [_ w1669]
              tunnel: w1642 -> [_ w1668]
              frame False {
                w1666 = 0.0 ("DeslocRA")
                n1419 = property on="Calagem" class="Bool"("Disabled"=u8 2) -> ()  [unwired: 2 in, 2 out]
              }
              frame True {
                n1420 = property on="Calagem" class="Bool"("Disabled"=u8 0) -> ()  [unwired: 2 in, 2 out]
              }
            }
            "DeslocRA" <- w1644
            "DeslocDEC" <- w1645
          }
          frame "GUIDER" {
            w1808 = 1 ("lower limit")
            w1809 = 400 ("upper limit")
            # "PROCESSO VARIABLE TRACKING"
            n1421 = case shown="True" "ClearRA" {
              frame False {
              }
              frame True {
                n1422 = local write "RA  RATE"(0 ("RA  RATE")) -> ()
              }
            }
            n1423 = call "Borda Subida.vi"("Entrada"="VARIABLE \nTRACKING") -> ("Boolean"=w1814:bool)  [unwired: 4 in]
            n1424 = call "Borda.vi"("Entrada"="VARIABLE \nTRACKING") -> ("Boolean"=w1813:bool)  [unwired: 4 in]
            n1425 = case shown="True" w1813 {
              frame False {
              }
              frame True {
                w1869 = "0" ("Set Point")
                w1875 = u16 2 items=["ZERO", "AH", "DEC", "TUBO", "CUP"] ("Controlador")
                w1872 = u16 1 items=["ZERO", "AH", "DEC", "TUBO", "CUP"] ("Controlador")
                # "Enviando ZERO o controlador para o movimento"
                n1426 = call "Monta Comando.vi"("Set Point"=w1869, "Comando"="GIRAR_VEL", "Dispositivo"="EIXO" ("Comando"), "Controlador"=w1872) -> ()  [unwired: 3 in, 3 out]
                n1427 = call "Monta Comando.vi"("Set Point"=w1869, "Comando"="GIRAR_VEL", "Dispositivo"="EIXO" ("Comando"), "Controlador"=w1875) -> ()  [unwired: 3 in, 3 out]
              }
            }
            n1428 = case shown="True" w1814 {
              frame False {
              }
              frame True {
                w1886 = u16 2 items=["ZERO", "AH", "DEC", "TUBO", "CUP"] ("Controlador")
                w1883 = u16 1 items=["ZERO", "AH", "DEC", "TUBO", "CUP"] ("Controlador")
                # "Enviar esses Valores \npara os controladores"
                n1429 = property on="Calagem" class="Bool"("Disabled"=u8 2) -> ()  [unwired: 2 in, 2 out]
                n1430 = Number To Decimal String(number="RA  RATE") -> (decimal integer string=w1879:string)  [unwired: 1 in]
                n1431 = Number To Decimal String(number="DEC RATE") -> (decimal integer string=w1877:string)  [unwired: 1 in]
                n1432 = call "Monta Comando.vi"("Set Point"=w1879, "Comando"="GIRAR_VEL", "Dispositivo"="EIXO" ("Comando"), "Controlador"=w1883) -> ()  [unwired: 3 in, 3 out]
                n1433 = call "Monta Comando.vi"("Set Point"=w1877, "Comando"="GIRAR_VEL", "Dispositivo"="EIXO" ("Comando"), "Controlador"=w1886) -> ()  [unwired: 3 in, 3 out]
              }
            }
            n1434 = case shown="True" "ClearDEC" {
              frame False {
              }
              frame True {
                n1435 = local write "DEC RATE"(0 ("RA  RATE")) -> ()
              }
            }
            n1436 = In Range and Coerce(upper limit=w1809, x="X STAR", lower limit=w1808) -> (In Range?=w1805:bool)  [unwired: 1 out]
            n1437 = In Range and Coerce(upper limit=w1809, x="Y STAR", lower limit=w1808) -> (In Range?=w1806:bool)  [unwired: 1 out]
            n1438 = In Range and Coerce(upper limit=w1809, x="X CENTER", lower limit=w1808) -> (In Range?=w1804:bool)  [unwired: 1 out]
            n1439 = In Range and Coerce(upper limit=w1809, x="Y CENTER", lower limit=w1808) -> (In Range?=w1803:bool)  [unwired: 1 out]
            n1440 = Compound Arithmetic op=AND(w1805, w1806, w1804, w1803, "XY CENTER") -> (w1807:bool)
            n1441 = case shown="True" w1807 {
              tunnel: "X STAR" -> [_ w1850]
              tunnel: "X CENTER" -> [_ w1849]
              tunnel: "Y STAR" -> [_ w1848]
              tunnel: "Y CENTER" -> [_ w1847]
              frame False {
              }
              frame True {
                # "MUDANÇA: IMPLEMENTADO MOV. XY DO GUIDER EM \n20-05-2011, MAS AINDA NÃO FOI TESTADO..."
                # "rad"
                # "Ativa o envio comando de deslocamento ao controlador"
                n1442 = global read "Global_Telescopio.vi" "guide_ang"() -> (w1838:string)
                n1443 = global read "Global_Telescopio.vi" "guide_nor"() -> (w1839:string)
                n1444 = global read "Global_Telescopio.vi" "guide_cas"() -> (w1846:string)
                n1445 = Subtract(x=w1850, y=w1849) -> (x-y=w1844:i32)
                n1446 = Subtract(x=w1848, y=w1847) -> (x-y=w1843:i32)
                n1447 = global read "Global_Telescopio.vi" "guide_esp"() -> (w1841:string)
                n1448 = To Double Precision Float(number=w1844) -> (double precision float=w1821:dbl)
                n1449 = To Double Precision Float(number=w1843) -> (double precision float=w1822:dbl)
                n1450 = Equal?(x=w1846, y="S") -> (x = y?=w1836:bool)
                n1451 = case shown="True" w1836 {
                  tunnel: w1839 -> [_ w1866]
                  tunnel: w1838 -> [_ w1863]
                  tunnel: [w1859 w1860] -> w1835
                  frame False {
                    # "Foco Coudé"
                    n1452 = call "AnguloFenda.vi"() -> ("AngFenda"=w1859:dbl)  [unwired: 3 in]
                  }
                  frame True {
                    # "Foco Cassegrain"
                    n1453 = Fract/Exp String To Number(use system decimal point (T)=FALSE, string=w1866) -> (number=w1861:dbl)  [unwired: 2 in, 1 out]
                    n1454 = Fract/Exp String To Number(use system decimal point (T)=FALSE, string=w1863) -> (number=w1862:dbl)  [unwired: 2 in, 1 out]
                    n1455 = Add(x=w1862, y=w1861) -> (x+y=w1860:dbl)
                  }
                }
                n1456 = Equal?(x=w1841, y="S") -> (x = y?=w1826:bool)
                n1457 = global write "Global_Telescopio.vi" "Correção Guider"("Habilita Movimento") -> ()
                n1458 = Multiply(x=0.01745329252 ("y"), y=w1835) -> (x*y=w1834:dbl)
                n1459 = Cosine(x=w1834) -> (cos(x)=w1823:dbl)
                n1460 = Sine(x=w1834) -> (sin(x)=w1824:dbl)
                n1461 = Multiply(x=w1821, y=w1823) -> (x*y=w1815:dbl)
                n1462 = Multiply(x=w1823, y=w1822) -> (x*y=w1820:dbl)
                n1463 = Multiply(x=w1822, y=w1824) -> (x*y=w1816:dbl)
                n1464 = Multiply(x=w1824, y=w1821) -> (x*y=w1819:dbl)
                n1465 = Subtract(x=w1820, y=w1819) -> (x-y=w1818:dbl)
                n1466 = Add(x=w1816, y=w1815) -> (x+y=w1817:dbl)
                n1467 = Less Than 0?(x=w1818) -> (x < 0?=w1832:bool)
                n1468 = Less Than 0?(x=w1817) -> (x < 0?=w1828:bool)
                n1469 = case shown="True" w1828 {
                  tunnel: w1826 -> [w1852 w1855]
                  tunnel: [w1851 w1856] -> w1825
                  frame False {
                    n1470 = Select(t="W" ("y"), s=w1852, f="E" ("y")) -> (s? t:f=w1851:string)
                  }
                  frame True {
                    n1471 = Select(t="E" ("y"), s=w1855, f="W" ("y")) -> (s? t:f=w1856:string)
                  }
                }
                n1472 = Select(t="S" ("y"), s=w1832, f="N" ("y")) -> (s? t:f=w1831:string)
                n1473 = Absolute Value(x=w1818) -> (abs(x)=w1829:dbl)
                n1474 = Absolute Value(x=w1817) -> (abs(x)=w1827:dbl)
                n1475 = global write "Global_Telescopio.vi" "guide_dir_we"(w1825) -> ()
                n1476 = global write "Global_Telescopio.vi" "guide_dir_ns"(w1831) -> ()
                n1477 = global write "Global_Telescopio.vi" "guide_dec"(w1829) -> ()
                n1478 = global write "Global_Telescopio.vi" "guide_asc"(w1827) -> ()
              }
            }
            "LED VAR TRACKING" <- "VARIABLE \nTRACKING"
          }
          frame "CALIBRATION" {
            # "Alterado dia 23/07/218"
            n1479 = disable-structure shown="Disabled" {
              frame Disabled {
              }
              frame Enabled {
              }
            }
            n1480 = event shown="[4] \"Coude\": Value Change" {
              selector: _ -> [_ _ _ _ _]
              dyn-events: _ -> [_ _ _ _ _]
              timeout: 10 -> [_ _ _ _ _]
              event Timeout {
                n1481 = event-data() -> ()  [unwired: 1 in, 2 out]
              }
              event "Weak": Value Change {
                w1892 = u16 6 items=["Alarme", "Atencao", "Erro", "Ocupado", "TBD", "LCB", "Trapeira", "Paravento", "DomoRap", "DomoCW", "DomoCCW", "TBD", "Em movimento", "TBD"] ("NomeStatus")
                n1482 = event-data() -> ("NewVal"=w1893:bool)  [unwired: 1 in, 5 out]
                n1483 = call "Bit Status CUP.vi"("NomeStatus"=w1892) -> ("StatBit"=w1891:bool)
                n1484 = case shown="False" w1891 {
                  tunnel: w1893 -> [w1900 _]
                  frame False {
                    w1894 = u16 4 items=["ZERO", "AH", "DEC", "TUBO", "CUP"] ("Controlador")
                    n1485 = case shown="True" w1900 {
                      tunnel: [w1901 TRUE ("WeakSel")] -> w1899
                      tunnel: [w1901 FALSE ("MediumSel")] -> w1897
                      tunnel: [0 2] -> w1896
                      tunnel: ["DESLIGAR" ("Comando") "LIGAR" ("Comando")] -> w1898
                      frame False {
                        w1901 = FALSE ("MediumSel")
                      }
                      frame True {
                        n1486 = local write "DOME"(FALSE) -> ()
                        n1487 = local write "StatShutter"("Busy to Close" ("Status")) -> ()
                      }
                    }
                    n1488 = property on="Coude" class="Bool (strict)"("DisabledEnum"=w1896) -> ()  [unwired: 2 in, 2 out]
                    n1489 = property on="WeakSel" class="Bool (strict)"("Value"=w1899) -> ()  [unwired: 2 in, 2 out]
                    n1490 = property on="CoudeSel" class="Bool (strict)"("Value"=w1897) -> ()  [unwired: 2 in, 2 out]
                    n1491 = property on="Strong" class="Bool (strict)"("Disabled"=w1896) -> ()  [unwired: 2 in, 2 out]
                    n1492 = property on="MediumSel" class="Bool (strict)"("Value"=w1897) -> ()  [unwired: 2 in, 2 out]
                    n1493 = property on="StrongSel" class="Bool (strict)"("Value"=w1897) -> ()  [unwired: 2 in, 2 out]
                    n1494 = property on="Medium" class="Bool (strict)"("Disabled"=w1896) -> ()  [unwired: 2 in, 2 out]
                    n1495 = call "Monta Comando.vi"("Comando"=w1898, "Dispositivo"="FLAT_WEAK", "Controlador"=w1894) -> ()  [unwired: 4 in, 3 out]
                  }
                  frame True {
                    w1910 = FALSE ("Weak")
